vi "Init.vi"(8 "error in (no error)":errorcluster) -> (0 "error out":errorcluster, 3 "View out":refnum<class "View.lvclass">)   [LabVIEW 2020, in "Page1.lvlib" / "View.lvclass"]
uses:
  View.lvclass
  View.lvclass/View.ctl
  Controller/Controller.lvclass
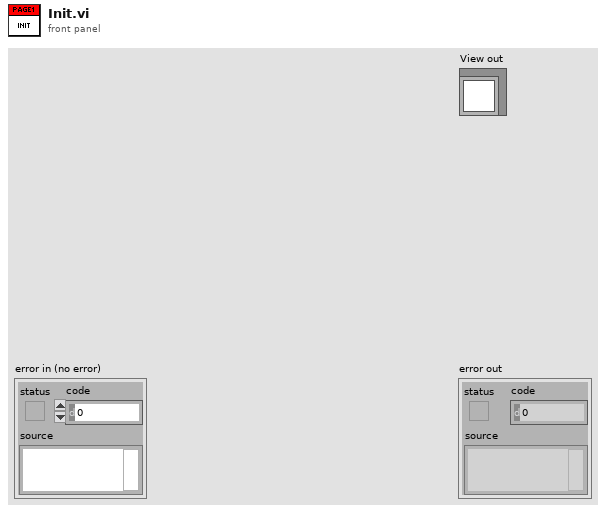
[diagram p1: front panel]
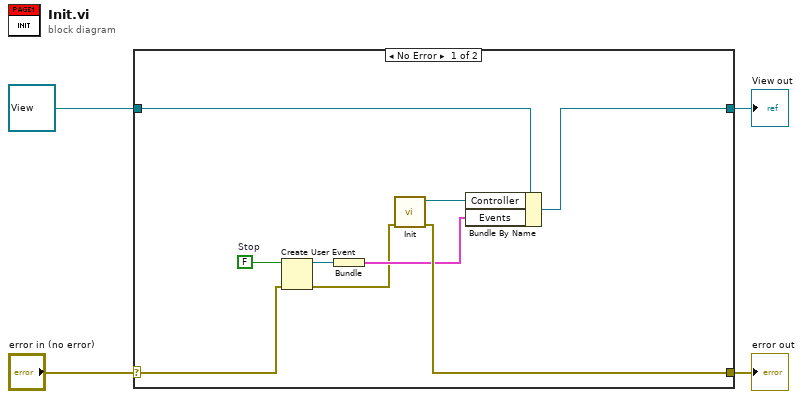
[diagram p0: block diagram]
diagram:
  n1 = case shown="No Error" "error in (no error)" {
    selector: "error in (no error)" -> [w7 w15]
    tunnel: [w10 w15] -> w3
    tunnel: [w12 w14] -> w2
    tunnel: refnum<class "View.lvclass"> refnum ("View in") -> [w13 w14]
    frame No Error {
      w9 = FALSE  # Stop
      n2 = Create User Event(user event datatype=w9, error in=w7) -> (user event=w8:refnum<user-event>, error out=w5:errorcluster)
      n3 = Bundle("Stop"=w8) -> (w6:cluster{"Stop":refnum<user-event>})  [unwired: 1 in]
      n4 = call "Init.vi"("error in (no error)"=w5) -> ("error out"=w10:errorcluster, "Controller out"=w11:refnum<class "Controller.lvclass">)  [unwired: 9 in]
      n5 = Bundle By Name(cluster=w13, "Controller"=w11, "Events"=w6) -> (w12:refnum<class "View.lvclass">)
    }
    frame Error {
    }
  }
  "error out" <- w3
  "View out" <- w2
